vi "SetSmallerGHigherPriority.vi"(10 "smaller g = higher priority":bool, 11 "priority queue in":refnum<class "NI_Robotics_Priority Queue.lvclass">) -> (3 "priority queue out":refnum<class "NI_Robotics_Priority Queue.lvclass">)   [LabVIEW 2017, in "NI_Robotics_Priority Queue.lvclass"]
uses:
  <vilib>/robotics/Navigation/shared/Priority Queue/NI_Robotics_Priority Queue.lvclass
  <vilib>/robotics/Navigation/shared/Priority Queue/NI_Robotics_Priority Queue.lvclass/NI_Robotics_Priority Queue.ctl
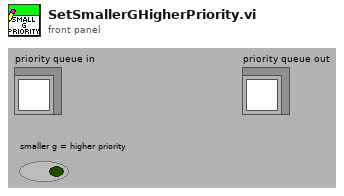
[diagram p1: front panel]
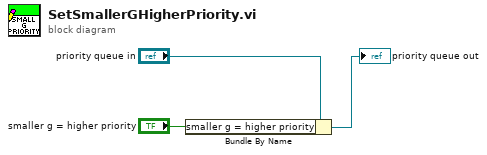
[diagram p0: block diagram]
diagram:
  n1 = Bundle By Name(cluster="priority queue in", "smaller g = higher priority"="smaller g = higher priority") -> (→"priority queue out":refnum<class "NI_Robotics_Priority Queue.lvclass">)
